vi "Create Chans.vi"(5 "New Section Name (none)":string, 7 "Type":T2=enum."Output", 8 "error in (no error)":errorcluster, 10 "Channels":T1[](array[typedef]), 11 "Section Ptr":T3 format="%.0x") -> (0 "error out":errorcluster, 3 "Section Ptr dup":T3 format="%.0x")   [LabVIEW 2012, in "PXImc System Explorer.lvlib"]
uses:
  PXImc System Explorer.lvlib
  <vilib>/NI Veristand/Custom Device API/Custom Device Item Ref.ctl
  <vilib>/NI Veristand/Custom Device API/Custom Device Channel Type.ctl
  Shared/Channel.ctl
  <vilib>/NI Veristand/Custom Device API/Custom Device Channel.ctl
  Shared/Constants.vi
  <vilib>/NI Veristand/Custom Device API/Custom Device API.lvlib
  Shared/PXImc Shared.lvlib
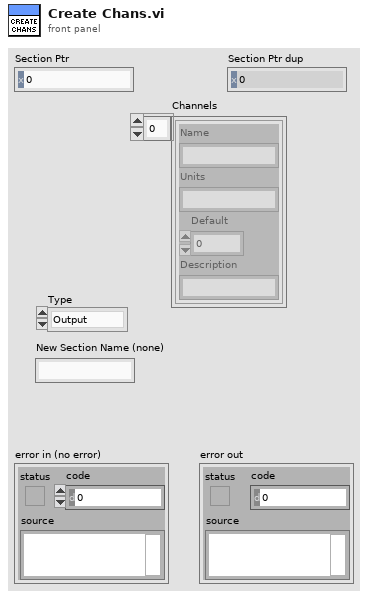
[diagram p1: front panel]
types:
  T1 = typedef "PXImc Shared.lvlib/Channel.ctl" = cluster{"Name":string, "Units":string, "Default":dbl, "Description":string}
  T2 = typedef "Custom Device API.lvlib/Custom Device Channel Type.ctl" = enum16{"Input", "Output"}
  T3 = typedef "Custom Device API.lvlib/Custom Device Item Ref.ctl" = u64
  T4 = typedef "Custom Device API.lvlib/Custom Device Channel.ctl" = cluster{"Type":T2, "Units":string, "Default Value":dbl, "Faultable":bool, "Scalable":bool}
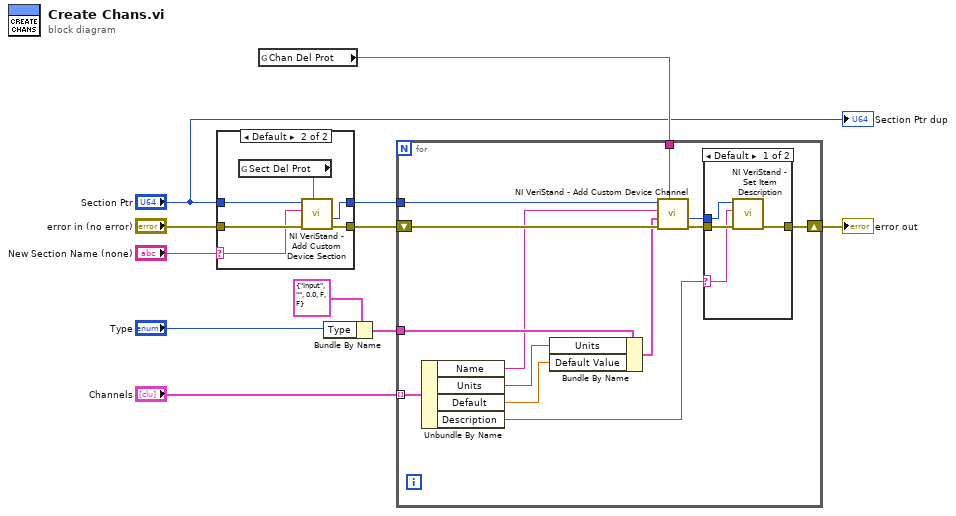
[diagram p0: block diagram]
diagram:
  n1 = case shown="Default" "New Section Name (none)" {
    selector: "New Section Name (none)" -> [_ w15]
    tunnel: "error in (no error)" -> [w13 w19]
    tunnel: "Section Ptr" -> [w12 w18]
    tunnel: [w13 w17] -> w4
    tunnel: [w12 w16] -> w3
    frame "" {
    }
    frame Default {
      n2 = global read "Constants.vi" "Sect Del Prot"() -> (w14:string)
      n3 = call <vilib>:"NI VeriStand - Add Custom Device Section.vi"("GUID (Default Section)"=w14, "error in (no error)"=w19, "Section Name"=w15, "Parent Ref in"=w18) -> ("error out"=w17:errorcluster, "Section Ptr"=w16:T3)  [unwired: 4 in, 2 out]
    }
  }
  n4 = global read "Constants.vi" "Chan Del Prot"() -> (w11:string)
  n5 = Bundle By Name(cluster=T4 {"Type"=enum."Input", "Units"="", "Default Value"=0.0, "Faultable"=FALSE, "Scalable"=FALSE} ("Channel"), "Type"="Type") -> (w5:T4)
  n6 = for {
    tunnel: w3 -> [w31]
    shift-right: [w27] -> w9
    shift-left: w4 -> [w32]
    tunnel: w5 -> [w30]
    tunnel: w11 -> [w28]
    tunnel: "Channels" -> [w24] mode=indexing
    n7 = Unbundle By Name(w24) -> ("Name"=w23:string, "Units"=w22:string, "Default"=w21:dbl, "Description"=w20:string)
    n8 = Bundle By Name(cluster=w30, "Units"=w22, "Default Value"=w21) -> (w29:T4)
    n9 = call <vilib>:"NI VeriStand - Add Custom Device Channel.vi"("GUID (Default Channel)"=w28, "error in (no error)"=w32, "Channel"=w29, "Channel Name"=w23, "Parent Ref in"=w31) -> ("error out"=w26:errorcluster, "Channel Ref"=w25:T3)  [unwired: 3 in, 2 out]
    n10 = case shown="Default" w20 {
      selector: w20 -> [w33 _]
      tunnel: [w35 w37] -> w27
      tunnel: w26 -> [w36 w37]
      tunnel: w25 -> [w34 _]
      frame Default {
        n11 = call <vilib>:"NI VeriStand - Set Item Description.vi"("error in (no error)"=w36, "Description"=w33, "Item Ref in"=w34) -> ("error out"=w35:errorcluster)  [unwired: 6 in, 2 out]
      }
      frame "" {
      }
    }
  }
  "error out" <- w9
  "Section Ptr dup" <- "Section Ptr"
